vi "Measure Element.vi"(8 "error in (no error)":errorcluster, 10 "Element (1: Element 1)":u16(ring)=1 items=["", "Element1", "Element2", "Element3", "Sigma"], 11 "VISA resource name":refnum<visa-resource-name>) -> (0 "error out":errorcluster, 2 "Array":string[][](array[string]), 3 "VISA resource name out":refnum<visa-resource-name>)   [LabVIEW 2013, in "Universal Power Meter.lvlib" / "Yokogawa WT2X0.lvlib" / "Yokogawa WT2X0.lvclass"]
uses:
  Yokogawa WT2X0.lvclass
  <instrlib>/Yokogawa WT200 Series/Yokogawa WT200 Series.lvlib
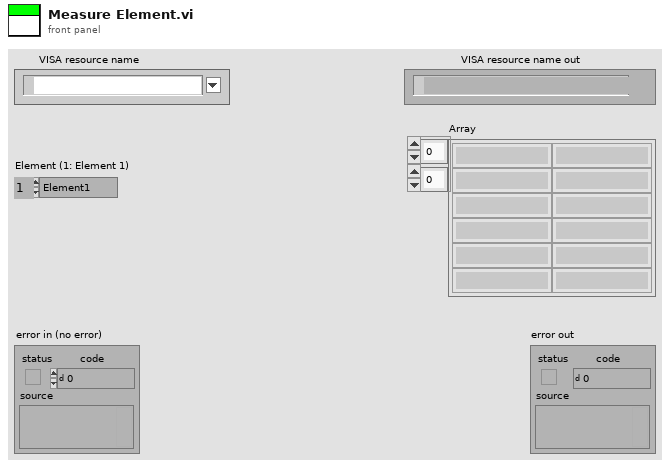
[diagram p1: front panel]
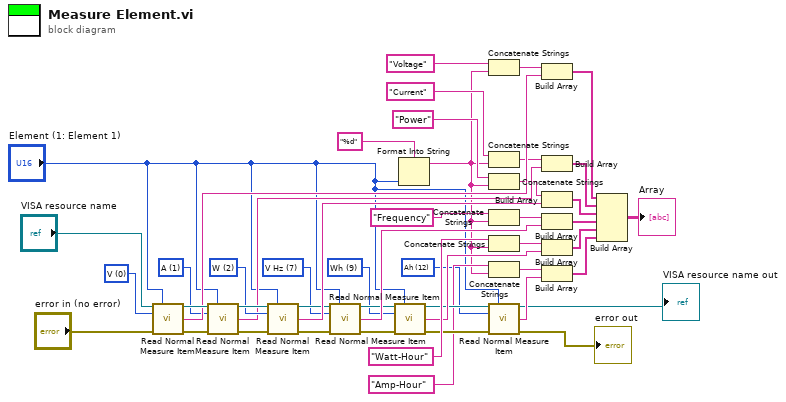
[diagram p0: block diagram]
diagram:
  w4 = u16 12 items=["V", "A", "W", "VA", "var", "PF", "deg", "V Hz", "A Hz", "Wh", "Wh+", "Wh-", "Ah", "Ah+", "Ah-", "Vpk", "Apk", "Math"] ("Measure Item (0: V)")
  w16 = u16 9 items=["V", "A", "W", "VA", "var", "PF", "deg", "V Hz", "A Hz", "Wh", "Wh+", "Wh-", "Ah", "Ah+", "Ah-", "Vpk", "Apk", "Math"] ("Measure Item (0: V)")
  w24 = u16 7 items=["V", "A", "W", "VA", "var", "PF", "deg", "V Hz", "A Hz", "Wh", "Wh+", "Wh-", "Ah", "Ah+", "Ah-", "Vpk", "Apk", "Math"] ("Measure Item (0: V)")
  w36 = u16 2 items=["V", "A", "W", "VA", "var", "PF", "deg", "V Hz", "A Hz", "Wh", "Wh+", "Wh-", "Ah", "Ah+", "Ah-", "Vpk", "Apk", "Math"] ("Measure Item (0: V)")
  w39 = u16 1 items=["V", "A", "W", "VA", "var", "PF", "deg", "V Hz", "A Hz", "Wh", "Wh+", "Wh-", "Ah", "Ah+", "Ah-", "Vpk", "Apk", "Math"] ("Measure Item (0: V)")
  w47 = u16 0 items=["V", "A", "W", "VA", "var", "PF", "deg", "V Hz", "A Hz", "Wh", "Wh+", "Wh-", "Ah", "Ah+", "Ah-", "Vpk", "Apk", "Math"] ("Measure Item (0: V)")
  n1 = call <instrlib>:"Read Normal Measure Item.vi"("VISA resource name"="VISA resource name", "Element (1: Element 1)"="Element (1: Element 1)", "Measure Item (0: V)"=w47, "error in (no error)"="error in (no error)") -> ("VISA resource name out"=w46:refnum<visa-resource-name>, "Measured Value"=w44:string, "error out"=w41:errorcluster)  [unwired: 8 in, 1 out]
  n2 = call <instrlib>:"Read Normal Measure Item.vi"("VISA resource name"=w46, "Element (1: Element 1)"="Element (1: Element 1)", "Measure Item (0: V)"=w39, "error in (no error)"=w41) -> ("VISA resource name out"=w38:refnum<visa-resource-name>, "Measured Value"=w33:string, "error out"=w37:errorcluster)  [unwired: 8 in, 1 out]
  n3 = call <instrlib>:"Read Normal Measure Item.vi"("VISA resource name"=w38, "Element (1: Element 1)"="Element (1: Element 1)", "Measure Item (0: V)"=w36, "error in (no error)"=w37) -> ("VISA resource name out"=w25:refnum<visa-resource-name>, "Measured Value"=w29:string, "error out"=w23:errorcluster)  [unwired: 8 in, 1 out]
  n4 = call <instrlib>:"Read Normal Measure Item.vi"("VISA resource name"=w25, "Element (1: Element 1)"="Element (1: Element 1)", "Measure Item (0: V)"=w24, "error in (no error)"=w23) -> ("VISA resource name out"=w18:refnum<visa-resource-name>, "Measured Value"=w21:string, "error out"=w17:errorcluster)  [unwired: 8 in, 1 out]
  n5 = call <instrlib>:"Read Normal Measure Item.vi"("VISA resource name"=w18, "Element (1: Element 1)"="Element (1: Element 1)", "Measure Item (0: V)"=w16, "error in (no error)"=w17) -> ("VISA resource name out"=w11:refnum<visa-resource-name>, "Measured Value"=w13:string, "error out"=w10:errorcluster)  [unwired: 8 in, 1 out]
  n6 = Format Into String(format string="%d", "Element (1: Element 1)") -> (resulting string=w7:string)  [unwired: 2 in, 1 out]
  n7 = Concatenate Strings("Voltage" ("string"), w7) -> (w43:string)
  n8 = Concatenate Strings("Current" ("string"), w7) -> (w35:string)
  n9 = Concatenate Strings("Power" ("string"), w7) -> (w27:string)
  n10 = Concatenate Strings("Frequency" ("string"), w7) -> (w20:string)
  n11 = Concatenate Strings("Watt-Hour" ("string"), w7) -> (w15:string)
  n12 = Concatenate Strings("Amp-Hour" ("string"), w7) -> (w8:string)
  n13 = call <instrlib>:"Read Normal Measure Item.vi"("VISA resource name"=w11, "Element (1: Element 1)"="Element (1: Element 1)", "Measure Item (0: V)"=w4, "error in (no error)"=w10) -> ("VISA resource name out"=→"VISA resource name out":refnum<visa-resource-name>, "Measured Value"=w6:string, "error out"=→"error out":errorcluster)  [unwired: 8 in, 1 out]
  n14 = Build Array(w43, w44) -> (w34:string[])
  n15 = Build Array(w35, w33) -> (w31:string[])
  n16 = Build Array(w27, w29) -> (w26:string[])
  n17 = Build Array(w20, w21) -> (w19:string[])
  n18 = Build Array(w15, w13) -> (w12:string[])
  n19 = Build Array(w8, w6) -> (w3:string[])
  n20 = Build Array(w34, w31, w26, w19, w12, w3) -> (→"Array":string[][])
